vi "Message type.vi"(11 "IInternalDoAbleMessage in":refnum<class "IGenericInternalMessage.lvclass">) -> (2 "Internal message type":T1, 3 "IInternalDoAbleMessage out":refnum<class "IGenericInternalMessage.lvclass">)   [LabVIEW 2020, in "wamplv.lvlib" / "IGenericInternalMessage.lvclass"]
uses:
  IGenericInternalMessage.lvclass
  TypeDefs/Internal message type.ctl
  wamplv.lvlib
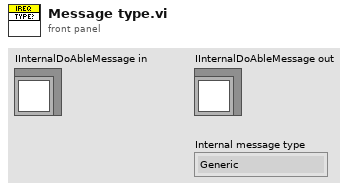
[diagram p1: front panel]
types:
  T1 = typedef "wamplv.lvlib/Internal message type.ctl" = enum16{"Generic", "Handle Result"}
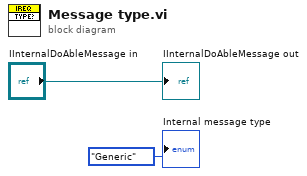
[diagram p0: block diagram]
diagram:
  "IInternalDoAbleMessage out" <- "IInternalDoAbleMessage in"
  "Internal message type" <- Internal_message_type."Generic" ("Internal message type")
